vi "Timebase conversion.vi"(8 "error in (no error)":errorcluster, 11 "PicoScope 3000a in":refnum<class "PicoScope 3000a.lvclass">) -> (0 "error out":errorcluster, 2 "Timebase":u32, 3 "PicoScope 3000a out":refnum<class "PicoScope 3000a.lvclass">)   [LabVIEW 2018, in "PicoScope 3000a.lvlib" / "PicoScope 3000a.lvclass"]
uses:
  PicoScope 3000a.lvclass
  PicoScope 3000a.lvclass/PicoScope 3000a.ctl
  <userlib>/_OpenG.lib/array/array.llb/Search 1D Array (Boolean)__ogtk.vi
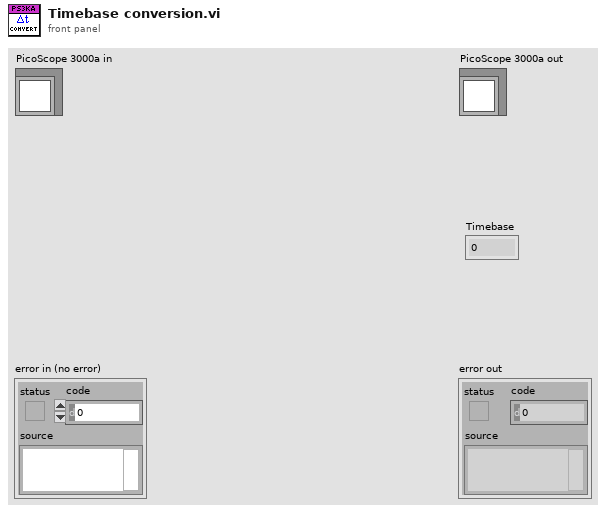
[diagram p1: front panel]
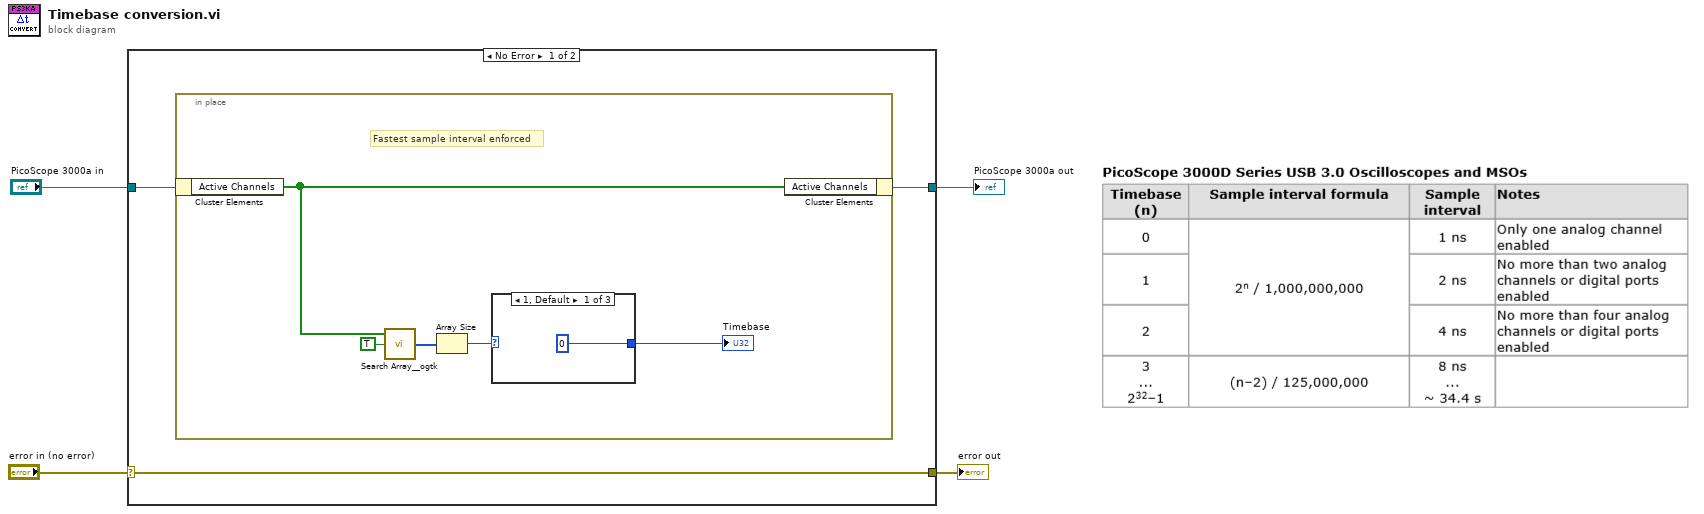
[diagram p0: block diagram]
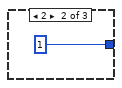
[diagram p2: hidden frame]
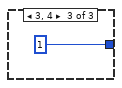
[diagram p3: hidden frame]
diagram:
  n1 = case shown="No Error" "error in (no error)" {
    selector: "error in (no error)" -> [w5 w17]
    tunnel: [w5 w17] -> w3
    tunnel: [w6 w16] -> w1
    tunnel: "PicoScope 3000a in" -> [w7 w16]
    frame No Error {
      n2 = in-place {
        # "Fastest sample interval enforced"
        n3 = in-place-cluster #1(w7) -> ("Active Channels"=w10:bool[])
        n4 = call-poly <userlib>:"Search Array__ogtk.vi"("Array"=w10, "Element Data"=TRUE) -> ("Indices of Elements"=w8:i32[])  [unwired: 7 in]
        n5 = Array Size(array=w8) -> (size(s)=w12:i32)
        n6 = case shown="1, Default" w12 {
          tunnel: [u32 0 u32 1 u32 1] -> w11
          frame 1, Default {
          }
          frame 2 {
          }
          frame 3, 4 {
          }
        }
        "Timebase" <- w11
        n7 = in-place-cluster #1("Active Channels"=w10) -> (w6:refnum<class "PicoScope 3000a.lvclass">)
      }
    }
    frame Error {
    }
  }
  "error out" <- w3
  "PicoScope 3000a out" <- w1
